vi "Save port config.vi"(8 "error in (no error)":errorcluster, 11 "Comm ports in":T1={"Piezo driver"="COM2", "Cam Session"="", "Arduino"="COM2"}) -> (0 "error out":errorcluster)   [LabVIEW 2020]
uses:
  Controls/Communication ports ---typedef.ctl
  <vilib>/userDefined/High Color/IMAQdx.ctl
  <vilib>/Utility/config.llb/Write Key (String).vi
  <vilib>/Utility/config.llb/NI_LVConfig.lvlib
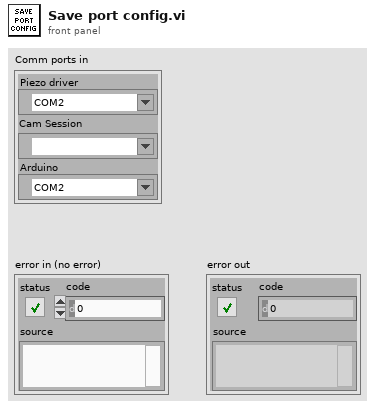
[diagram p1: front panel]
types:
  T1 = typedef "Communication ports ---typedef.ctl" = cluster{"Piezo driver":refnum<visa-resource-name>, "Cam Session":T2, "Arduino":refnum<visa-resource-name>}
  T2 = typedef "IMAQdx.ctl" = refnum<k21>
  T3 = typedef "NI_LVConfig.lvlib/Config Data RefNum.ctl" = refnum<k1>
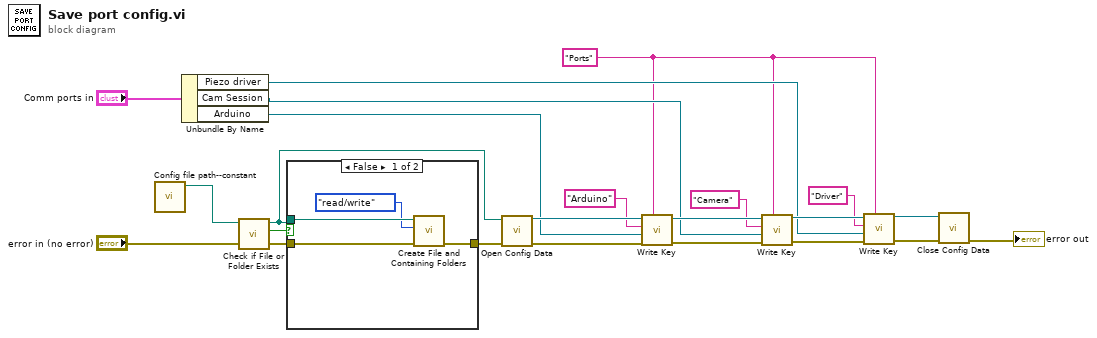
[diagram p0: block diagram]
diagram:
  w1 = "Ports" ("section")
  n1 = call "Config file path--constant.vi"() -> ("appended path"=w23:path)  [unwired: 11 in]
  n2 = Unbundle By Name("Comm ports in") -> ("Piezo driver"=w2:refnum<visa-resource-name>, "Cam Session"=w9:T2, "Arduino"=w13:refnum<visa-resource-name>)
  n3 = call <vilib>:"Check if File or Folder Exists.vi"("error in (no error)"="error in (no error)", "path"=w23) -> ("error out"=w21:errorcluster, "file or folder exists?"=w22:bool, "dup path"=w19:path)  [unwired: 7 in]
  n4 = case shown="False" w22 {
    tunnel: w19 -> [w27 _]
    tunnel: w21 -> [w26 w28]
    tunnel: [w24 w28] -> w20
    frame False {
      n5 = call <vilib>:"Create File and Containing Folders.vi"("error in (no error)"=w26, "access"=enum16{"read/write", "read-only", "write-only"}."read/write", "file path"=w27) -> ("error out"=w24:errorcluster)  [unwired: 7 in, 1 out]
    }
    frame True {
    }
  }
  n6 = call <vilib>:"Open Config Data.vi"("error in (no error)"=w20, "configuration file path"=w19) -> ("error out"=w17:errorcluster, "refnum"=w16:T3)  [unwired: 7 in, 1 out]
  n7 = call-poly <vilib>:"Write Key.vi"("section"=w1, "error in (no error)"=w17, "value"=w13, "key"="Arduino", "refnum"=w16) -> ("error out"=w12:errorcluster, "refnum out"=w11:T3)  [unwired: 4 in, 1 out]
  n8 = call-poly <vilib>:"Write Key.vi"("section"=w1, "error in (no error)"=w12, "value"=w9, "key"="Camera", "refnum"=w11) -> ("error out"=w8:errorcluster, "refnum out"=w7:T3)  [unwired: 4 in, 1 out]
  n9 = call-poly <vilib>:"Write Key.vi"("section"=w1, "error in (no error)"=w8, "value"=w2, "key"="Driver", "refnum"=w7) -> ("error out"=w6:errorcluster, "refnum out"=w5:T3)  [unwired: 4 in, 1 out]
  n10 = call <vilib>:"Close Config Data.vi"("error in (no error)"=w6, "refnum"=w5) -> ("error out"=→"error out":errorcluster)  [unwired: 8 in, 1 out]
